vi "Get Camera Image.vi"(10 "index":i32, 11 "output cluster":T2) -> (3 "Refnum out":T1)   [LabVIEW 2015]
uses:
  <vilib>/vision/Image Controls.llb/IMAQ Image.ctl
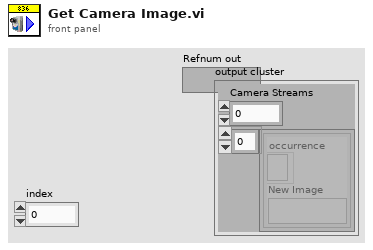
[diagram p1: front panel]
types:
  T1 = typedef "IMAQ Image.ctl" = refnum<image>
  T2 = cluster{"Camera Streams":i32, cluster{"occurrence":refnum<k4>, "New Image":T1}[]}
  T3 = cluster{"occurrence":refnum<k4>, "New Image":T1}[]
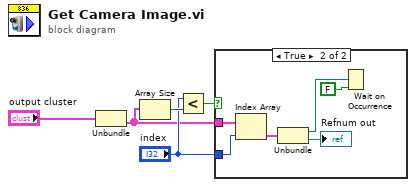
[diagram p0: block diagram]
diagram:
  n1 = Unbundle("output cluster") -> (w1:T3)  [unwired: 1 out]
  n2 = Array Size(array=w1) -> (size(s)=w4:i32)
  n3 = Less?(x="index", y=w4) -> (x < y?=w5:bool)
  n4 = case shown="True" w5 {
    tunnel: w1 -> [_ w8]
    tunnel: "index" -> [_ w7]
    frame False {
    }
    frame True {
      n5 = Index Array(array=w8, index=w7) -> (element=w10:cluster{"occurrence":refnum<k4>, "New Image":T1})
      n6 = Unbundle(w10) -> ("occurrence"=w9:refnum<k4>, "New Image"=→"Refnum out":T1)
      n7 = Wait on Occurrence(1:FALSE ("ignore previous (T)"), 2:w9) -> ()  [unwired: 1 in, 1 out]
    }
  }
